vi "Set Remote PID Setpoints Continuously.vi"(7 "VISA resource name":refnum<visa-resource-name>, 8 "error in":errorcluster, 10 "Remote Setpoint":i16[](array[numeric]), 11 "Unit Addresses":u8[](array[numeric])) -> (0 "error in (no error)":errorcluster)   [LabVIEW 2011, in "Owlstone GEN-SYS.lvclass"]
uses:
  Owlstone GEN-SYS.lvclass
  <instrlib>/Eurotherm 32xx Series/Eurotherm 32xx Series.lvlib
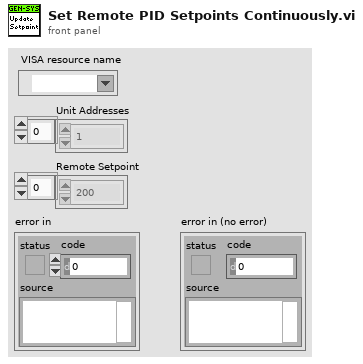
[diagram p1: front panel]
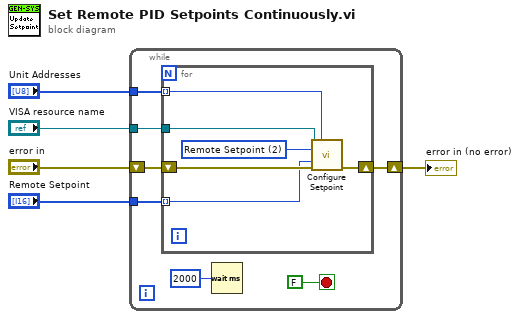
[diagram p0: block diagram]
diagram:
  n1 = while {
    tunnel: "Unit Addresses" -> [w11]
    tunnel: "Remote Setpoint" -> [w10]
    shift-right: [w8] -> w2
    shift-left: "error in" -> [w12]
    tunnel: "VISA resource name" -> [w6]
    stop <- FALSE stop-if-true
    n2 = for {
      tunnel: w11 -> [w16] mode=indexing
      tunnel: w10 -> [w15] mode=indexing
      shift-right: [w14] -> w8
      shift-left: w12 -> [w17]
      tunnel: w6 -> [w13]
      w18 = u8 2 items=["Setpoint 1", "Setpoint 2", "Remote Setpoint", "Target Setpoint"] ("Setpoint (0: Setpoint 1)")
      n3 = call <instrlib>:"Configure Setpoint.vi"("VISA resource name"=w13, "Unit Address (1)"=w16, "Setpoint (0: Setpoint 1)"=w18, "Setpoint Value (0)"=w15, "error in (no error)"=w17) -> ("error out"=w14:errorcluster)  [unwired: 9 in, 1 out]
    }
    n4 = Wait (ms)(milliseconds to wait=u32 2000) -> ()  [unwired: 1 out]
  }
  "error in (no error)" <- w2
